vi "Space Controls.vi"(8 "error in":errorcluster, 11 "Controls in":refnum<vi>[](array[refnum])) -> (0 "error out":errorcluster, 1 "Max right location":i32, 3 "Controls out":refnum<vi>[](array[refnum]))   [LabVIEW 2011, in "Align To Connector.lvlib"]
uses:
  Align To Connector.lvlib
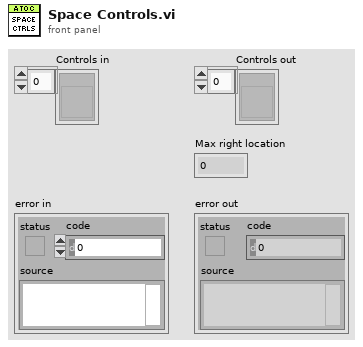
[diagram p1: front panel]
types:
  T1 = typedef "LVRectTypeDef.ctl" = cluster{"Left":i16, "Top":i16, "Right":i16, "Bottom":i16}
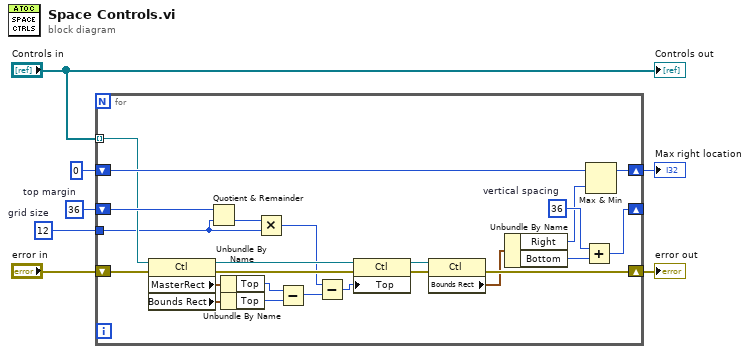
[diagram p0: block diagram]
diagram:
  w1 = 12  # grid size
  w7 = 36  # top margin
  n1 = for {
    tunnel: "Controls in" -> [w19] mode=indexing
    shift-right: [w30] -> _
    shift-left: w7 -> [w28]
    shift-right: [w26] -> w6
    shift-left: "error in" -> [w20]
    shift-right: [w25] -> w3
    shift-left: 0 -> [w24]
    tunnel: w1 -> [w8]
    w31 = 36  # vertical spacing
    n2 = property class="Ctl"(reference=w19, error in=w20) -> (reference out=w18:refnum<vi>, error out=w17:errorcluster, "MasterRect"=w16:T1, "Bounds Rect"=w15:T1)
    n3 = Quotient & Remainder(x=w28, y=w8) -> (floor(x/y)=w9:i32)  [unwired: 1 out]
    n4 = Unbundle By Name(w16) -> ("Top"=w14:i16)
    n5 = Unbundle By Name(w15) -> ("Top"=w13:i16)
    n6 = Multiply(x=w9, y=w8) -> (x*y=w10:i32)
    n7 = Subtract(x=w14, y=w13) -> (x-y=w11:i16)
    n8 = Subtract(x=w10, y=w11) -> (x-y=w12:i32)
    n9 = property class="Ctl"(reference=w18, error in=w17, "Top"=w12) -> (reference out=w29:refnum<vi>, error out=w27:errorcluster)
    n10 = property class="Ctl"(reference=w29, error in=w27) -> (error out=w26:errorcluster, "Bounds Rect"=w23:T1)  [unwired: 1 out]
    n11 = Unbundle By Name(w23) -> ("Right"=w22:i16, "Bottom"=w21:i16)
    n12 = Add(x=w31, y=w21) -> (x+y=w30:i32)
    n13 = Max & Min(x=w24, y=w22) -> (max(x,y)=w25:i32)  [unwired: 1 out]
  }
  "Max right location" <- w3
  "error out" <- w6
  "Controls out" <- "Controls in"
